vi "VectorLength.vi"(1 "VectorIn":T1) -> (0 "VectorLength":dbl)   [LabVIEW 2018, in "ArgosLib.lvlib"]
uses:
  ArgosLib.lvlib
  Path Planning/TypeDefs/Point2D.ctl
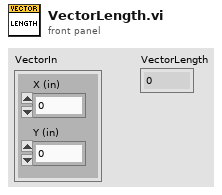
[diagram p1: front panel]
types:
  T1 = typedef "ArgosLib.lvlib/Point2D.ctl" = cluster{"X (in)":dbl, "Y (in)":dbl}
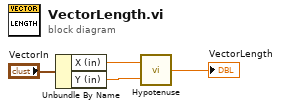
[diagram p0: block diagram]
diagram:
  n1 = Unbundle By Name("VectorIn") -> ("X (in)"=w3:dbl, "Y (in)"=w2:dbl)
  n2 = call "Hypotenuse.vi"("Y"=w2, "X"=w3) -> ("Hypotenuse"=→"VectorLength":dbl)
